vi "Compute alpha(beta) Plot.vi"(8 "Error In":errorcluster, 10 "Phasor Parameters":T1={"Display Parameters"={"# Points"=0, "Ramp Type"=enum."Linear", "Type of Series"=enum."1-Exp Decays", "Min tau"=0.0, "Max tau"=0.0, "Include 0"=FALSE, "Include Infinity"=FALSE}, "Phasor Parameters"={"Harmonic frequency"=0.0, "Use f* = 1/D Frequency"=FALSE, "Calibrated Phasor"=FALSE, "Calibration Lifetime"=1e-09, "Phasor Calculation"=enum."Direct Sum", "SEPL Type"=enum."UC", "# Gates"=1.0, "Square Gate Width"=1e-09, "Show Ticks"=FALSE}, "Decay & IRF Parameters"={"Lifetime"=0.0, "IRF Offset"=0.0, "Laser Period"=0.0, "Normalized Decays"=FALSE, "IRF Model"=enum."Dirac", "IRF Parameter 1"=0.0}, "Gate Parameters"={"First Gate Start"=0.0, "Use Gate Center"=FALSE, "Gate Width"=0.0, "Gate Step"=0.0, "# Gates"=0.0, "Gate Type"=enum."Square", "Edge Width"=0.0, "Top Slope"=0.0, "Reversed Sawtooth?"=FALSE, "Analytical Computation"=FALSE, "Tolerance"=1.0, "Integration"=enum."Item 0", "# Steps"=1.0, "Type of User-defined Function"=enum."Gate"}, "Detector Parameters"={"Frames/Image"=0, "Gates/Frame"=0, "Bits/Frame"=0, "Multiplicity"=0, "Incident Signal"=0.0}} {"Detector Parameters"."Frames/Image" min=1; "Detector Parameters"."Multiplicity" min=0; "Detector Parameters"."Bits/Frame" min=1; "Detector Parameters"."Gates/Frame" min=1; "Gate Parameters"."# Steps" min=0.0; "Gate Parameters"."Tolerance" min=0.0; "Gate Parameters"."Top Slope" min=0.0; "Gate Parameters"."Edge Width" min=0.0; "Gate Parameters"."Gate Step" min=0.0; "Gate Parameters"."# Gates" min=0.0 step=1.0; "Gate Parameters"."Gate Width" min=0.0; "Decay & IRF Parameters"."Lifetime" min=0.0; "Decay & IRF Parameters"."Laser Period" min=0.0; "Phasor Parameters"."Square Gate Width" min=0.0; "Phasor Parameters"."# Gates" min=0.0; "Phasor Parameters"."Calibration Lifetime" min=0.0; "Phasor Parameters"."Harmonic frequency" min=0.0; "Display Parameters"."Min tau" min=0.0; "Display Parameters"."Max tau" min=0.0; "Display Parameters"."# Points" min=1 step=1}, 11 "alpha(beta) Graph Refnum":refnum<vi>) -> (0 "Error Out":errorcluster, 2 "Max Lifetime":dbl[unit], 3 "Min Lifetime":dbl[unit])   [LabVIEW 2019]
uses:
  Pseudo Phasor Parameters.ctl
  Phasor Explorer Display Parameters.ctl
  Type of Series.ctl
  Phasor Explorer Phasor Parameters.ctl
  Phasor Calculation Type.ctl
  Phasor Type.ctl
  Phasor Explorer Decay Parameters.ctl
  IRF Model.ctl
  Phasor Explorer Gate Parameters.ctl
  Gate Type.ctl
  Phasor Explorer Detector Parameters.ctl
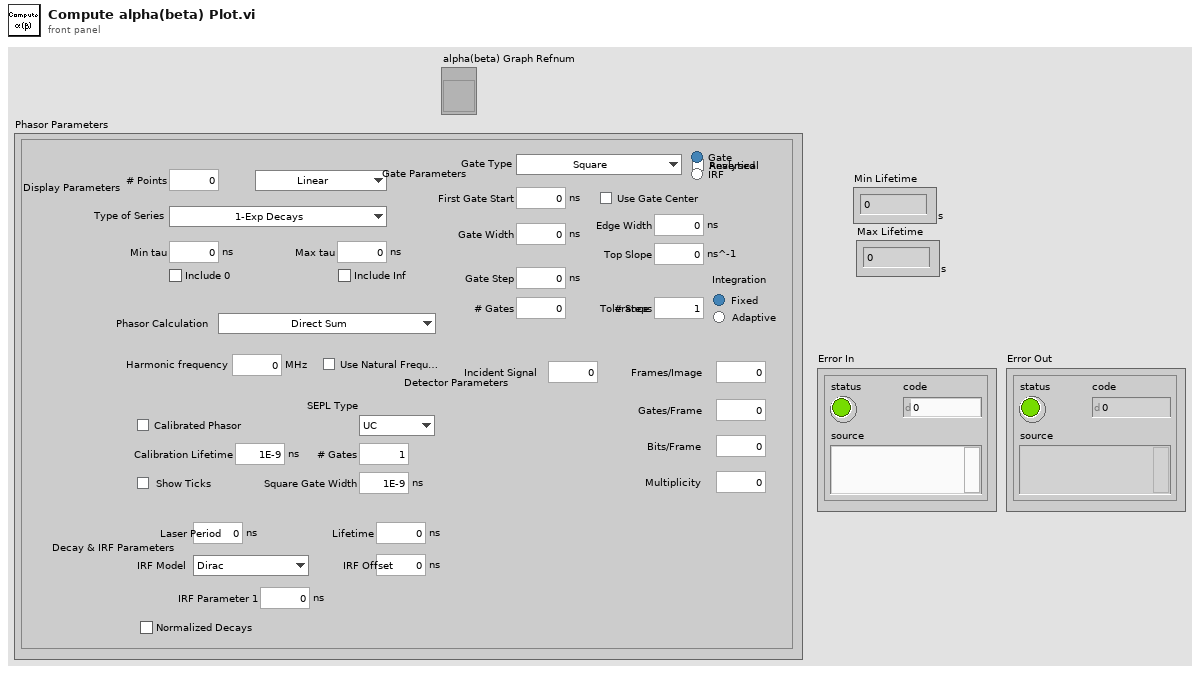
[diagram p1: front panel]
types:
  T1 = typedef "Pseudo Phasor Parameters.ctl" = cluster{"Display Parameters":T2, "Phasor Parameters":T4, "Decay & IRF Parameters":T7, "Gate Parameters":T9, "Detector Parameters":T11}
  T2 = typedef "Phasor Explorer Display Parameters.ctl" = cluster{"# Points":i32, "Ramp Type":enum16{"Linear", "Logarithmic"}, "Type of Series":T3, "Min tau":dbl[unit], "Max tau":dbl[unit], "Include 0":bool, "Include Infinity":bool}
  T3 = typedef "Type of Series.ctl" = enum16{"1-Exp Decays", "Linear Combination of 1-Exp"}
  T4 = typedef "Phasor Explorer Phasor Parameters.ctl" = cluster{"Harmonic frequency":dbl[unit], "Use f* = 1/D Frequency":bool, "Calibrated Phasor":bool, "Calibration Lifetime":dbl[unit], "Phasor Calculation":T5, "SEPL Type":T6, "# Gates":dbl, "Square Gate Width":dbl[unit], "Show Ticks":bool}
  T5 = typedef "Phasor Calculation Type.ctl" = enum16{"Direct Sum", "Analytical Formula"}
  T6 = typedef "Phasor Type.ctl" = enum16{"UC", "L_N", "L_N[W]"}
  T7 = typedef "Phasor Explorer Decay Parameters.ctl" = cluster{"Lifetime":dbl[unit], "IRF Offset":dbl[unit], "Laser Period":dbl[unit], "Normalized Decays":bool, "IRF Model":T8, "IRF Parameter 1":dbl[unit]}
  T8 = typedef "IRF Model.ctl" = enum16{"Dirac", "Exponential"}
  T9 = typedef "Phasor Explorer Gate Parameters.ctl" = cluster{"First Gate Start":dbl[unit], "Use Gate Center":bool, "Gate Width":dbl[unit], "Gate Step":dbl[unit], "# Gates":dbl, "Gate Type":T10, "Edge Width":dbl[unit], "Top Slope":dbl[unit], "Reversed Sawtooth?":bool, "Analytical Computation":bool, "Tolerance":dbl, "Integration":enum32{"Item 0", "Item 1"}, "# Steps":dbl, "Type of User-defined Function":enum32{"Gate", "IRF"}}
  T10 = typedef "Gate Type.ctl" = enum16{"Square", "Finite Edge Square", "Finite Edge, Tilted Top Square", "Triangle", "Sawtooth", "User-defined"}
  T11 = typedef "Phasor Explorer Detector Parameters.ctl" = cluster{"Frames/Image":i32, "Gates/Frame":i32, "Bits/Frame":i32, "Multiplicity":i32, "Incident Signal":dbl}
  T12 = typedef "Gate Definitions.ctl" = cluster{"First Gate: t1":ext, "Gate Width: W":ext, "Gate Step: d":ext, "# Gates: G":ext, "Use Gate Center":bool, "Frames/Image: F":i32, "Gates/Frame: L":i32, "Bits/Frame: q":i32, "Multiplicity: p":i32, "Gate Type":T10, "Gate Edge s":ext, "Gate Top Slope":ext, "Reversed Sawtooth?":bool, "Computation":bool, "User-defined Gate":T13, "Tolerance":ext, "Integration":enum32{"Item 0", "Item 1"}, "# Steps":ext, "Type of User-defined Function":enum32{"Gate", "IRF"}}
  T13 = typedef "XY Plot Data.ctl" = cluster{"X Array":dbl[], "Y Array":dbl[]}
  T14 = typedef "Decay Definiton.ctl" = cluster{"offset: t0":ext, "period: T":ext, "lifetime: tau":ext, "Incident Signal: I":ext, "Normalized Decays":bool, "IRF Model":T8, "IRF Parameter 1":ext}
  T15 = typedef "Phasor (g, s).ctl" = cluster{"g":dbl, "s":dbl}
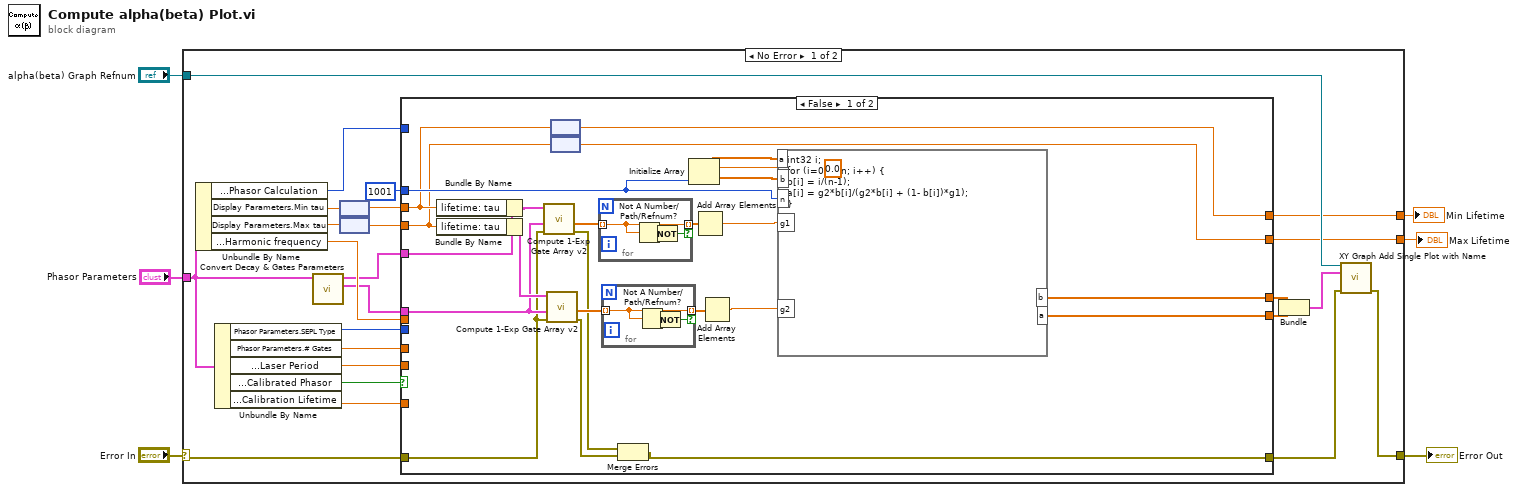
[diagram p0: block diagram]
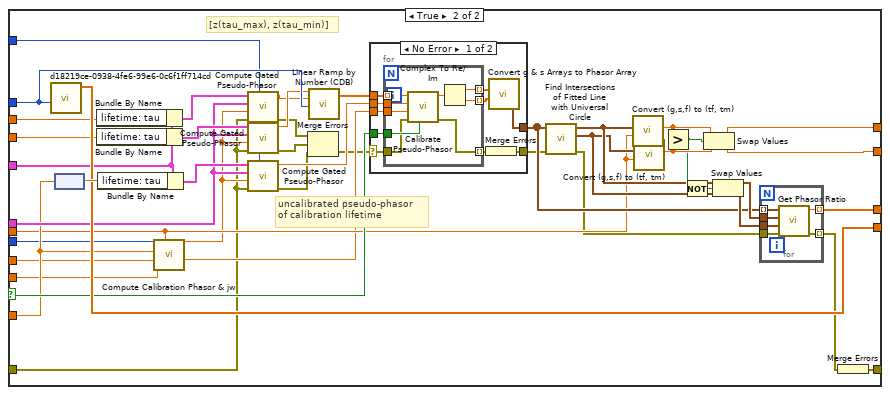
[diagram p2: hidden frame]
diagram:
  n1 = case shown="No Error" "Error In" {
    selector: "Error In" -> [w8 w130]
    tunnel: "Phasor Parameters" -> [w15 _]
    tunnel: "alpha(beta) Graph Refnum" -> [w28 _]
    tunnel: [w27 w130] -> w3
    tunnel: [w19 _] -> w2
    tunnel: [w18 _] -> w1
    frame No Error {
      n2 = Unbundle By Name(w15) -> ("Phasor Parameters.Phasor Calculation"=w12:T5, "Display Parameters.Min tau"=w29:dbl[unit], "Display Parameters.Max tau"=w30:dbl[unit], "Phasor Parameters.Harmonic frequency"=w20:dbl[unit])
      n3 = Unbundle By Name(w15) -> ("Phasor Parameters.SEPL Type"=w11:T6, "Phasor Parameters.# Gates"=w10:dbl, "Decay & IRF Parameters.Laser Period"=w9:dbl[unit], "Phasor Parameters.Calibrated Phasor"=w14:bool, "Phasor Parameters.Calibration Lifetime"=w13:dbl[unit])
      n4 = call "Convert Decay & Gates Parameters.vi"("Phasor Parameters"=w15) -> ("Gates Definitions"=w16:T12, "Decay Definition"=w17:T14)  [unwired: 9 in]
      n5 = node(w29) -> (w25:dbl)
      n6 = node(w30) -> (w24:dbl)
      n7 = case shown="False" w14 {
        selector: w14 -> [_ w80]
        tunnel: w17 -> [w52 w88]
        tunnel: w25 -> [w42 w89]
        tunnel: w24 -> [w40 w87]
        tunnel: w16 -> [w50 w84]
        tunnel: [w45 w91] -> w23
        tunnel: [w44 w90] -> w22
        tunnel: 1001 ("dimension size") -> [w43 w83]
        tunnel: w20 -> [_ w74]
        tunnel: [w41 w99] -> w19
        tunnel: [w39 w98] -> w18
        tunnel: w13 -> [_ w75]
        tunnel: w12 -> [_ w76]
        tunnel: w11 -> [_ w72]
        tunnel: w10 -> [_ w71]
        tunnel: w9 -> [_ w70]
        tunnel: w8 -> [w34 w68]
        tunnel: [w32 w62] -> w7
        frame False {
          n8 = Bundle By Name(cluster=w52, "lifetime: tau"=w42) -> (w51:T14)
          n9 = Bundle By Name(cluster=w52, "lifetime: tau"=w40) -> (w53:T14)
          n10 = call "Compute 1-Exp Gate Array v2.vi"("Error In"=w34, "Gates Definitions"=w50, "Decay Definition"=w51) -> ("Error Out"=w31:errorcluster, "Gate Image Array"=w38:ext[])  [unwired: 4 in, 3 out]
          n11 = call "Compute 1-Exp Gate Array v2.vi"("Error In"=w34, "Gates Definitions"=w50, "Decay Definition"=w53) -> ("Error Out"=w33:errorcluster, "Gate Image Array"=w36:ext[])  [unwired: 4 in, 3 out]
          n12 = node(w42) -> (w41:dbl[unit])
          n13 = node(w40) -> (w39:dbl[unit])
          n14 = for {
            tunnel: w38 -> [w59] mode=indexing
            tunnel: [w59] -> w37 mode=indexing if=w57
            n15 = Not A Number/Path/Refnum?(number/path/refnum=w59) -> (NaN/Path/Refnum?=w58:bool)
            n16 = Not(x=w58) -> (.not. x?=w57:bool)
          }
          n17 = for {
            tunnel: w36 -> [w56] mode=indexing
            tunnel: [w56] -> w35 mode=indexing if=w54
            n18 = Not A Number/Path/Refnum?(number/path/refnum=w56) -> (NaN/Path/Refnum?=w55:bool)
            n19 = Not(x=w55) -> (.not. x?=w54:bool)
          }
          n20 = Merge Errors(w31, w33) -> (w32:errorcluster)
          n21 = Initialize Array(0.0 ("element"), w43) -> (w46:dbl[])
          n22 = Add Array Elements(numeric array=w37) -> (sum=w49:ext)
          n23 = Add Array Elements(numeric array=w35) -> (sum=w48:ext)
          n24 = formula code="int32 i;\nfor (i=0; i<n; i++) {\nb[i] = i/(n-1);\na[i] = g2*b[i]/(g2*b[i] + (1- b[i])*g1);\n}"("g1"=w49, "g2"=w48, "b"=w46, "a"=w46, "n"=w43) -> ("b"=w45:dbl[], "a"=w44:dbl[])
        }
        frame True {
          # "[z(tau_max), z(tau_min)]"
          # "uncalibrated pseudo-phasor\nof calibration lifetime"
          n25 = call "d18219ce-0938-4fe6-99e6-0c6f1ff714cd.vi"("# Steps (1)"=w83) -> ("Ramp"=w90:dbl[])  [unwired: 9 in, 1 out]
          n26 = node(w75) -> (w102:dbl)
          n27 = Bundle By Name(cluster=w88, "lifetime: tau"=w89) -> (w86:T14)
          n28 = Bundle By Name(cluster=w88, "lifetime: tau"=w87) -> (w85:T14)
          n29 = Bundle By Name(cluster=w88, "lifetime: tau"=w102) -> (w103:T14)
          n30 = call "Compute Calibration Phasor & jw.vi"("Harmonic frequency"=w74, "Laser Period"=w70, "# Gates"=w71, "Calibration Lifetime"=w75, "Calibration Phasor Type"=w72) -> ("z (tau_cal)"=w69:cdb, "i 2 pi f (GHz)"=w73:cdb)  [unwired: 5 in]
          n31 = call "Compute Gated Pseudo-Phasor.vi"("Phasor Calculation Type"=w76, "Error In"=w68, "j 2 pi f"=w73, "Gates Definitions"=w84, "Decay Definition"=w86) -> ("Error Out"=w67:errorcluster, "phasor"=w78:cxt)  [unwired: 4 in, 1 out]
          n32 = call "Compute Gated Pseudo-Phasor.vi"("Phasor Calculation Type"=w76, "Error In"=w68, "j 2 pi f"=w73, "Gates Definitions"=w84, "Decay Definition"=w85) -> ("Error Out"=w66:errorcluster, "phasor"=w79:cxt)  [unwired: 4 in, 1 out]
          n33 = call "Compute Gated Pseudo-Phasor.vi"("Phasor Calculation Type"=w76, "Error In"=w68, "j 2 pi f"=w73, "Gates Definitions"=w84, "Decay Definition"=w103) -> ("Error Out"=w65:errorcluster, "phasor"=w81:cxt)  [unwired: 4 in, 1 out]
          n34 = Merge Errors(w67, w66, w65) -> (w61:errorcluster)
          n35 = call "Linear Ramp by Number (CDB).vi"("# Steps"=w83, "End"=w78, "Start"=w79) -> ("Ramp"=w82:cdb[])  [unwired: 7 in, 1 out]
          n36 = case shown="No Error" w61 {
            selector: w61 -> [w106 w123]
            tunnel: [w113 _] -> w92
            tunnel: w82 -> [w112 _]
            tunnel: w81 -> [w111 _]
            tunnel: w80 -> [w108 _]
            tunnel: w69 -> [w107 _]
            tunnel: [w104 w123] -> w60
            frame No Error {
              n37 = for {
                tunnel: w112 -> [w121] mode=indexing
                tunnel: w111 -> [w120]
                tunnel: w107 -> [w119]
                tunnel: [w118] -> w110 mode=indexing
                tunnel: [w117] -> w109 mode=indexing
                tunnel: w108 -> [w116]
                tunnel: w106 -> [w115]
                tunnel: [w114] -> w105 mode=indexing
                n38 = call "Calibrate Pseudo-Phasor.vi"("Calibrated Phasor"=w116, "Error In"=w115, "Target Phasor"=w119, "Calibration Pseudo-Phasor"=w120, "Pseudo-Phasor in"=w121) -> ("Error Out"=w114:errorcluster, "Pseudo-Phasor out"=w122:cxt)  [unwired: 5 in]
                n39 = Complex To Re/Im(x + iy=w122) -> (x=w118:ext, y=w117:ext)
              }
              n40 = Merge Errors(w105) -> (w104:errorcluster)
              n41 = call "Convert g & s Arrays to Phasor Array.vi"("s"=w109, "g"=w110) -> ("Phasor Array"=w113:T15[])  [unwired: 8 in]
            }
            frame Error {
            }
          }
          n42 = call "Find Intersections of Fitted Line with Universal Circle.vi"("Error In"=w60, "Phasor Array"=w92) -> ("Error Out"=w64:errorcluster, "Point 2"=w95:cluster{"x":dbl, "y":dbl}, "Point 1"=w96:cluster{"x":dbl, "y":dbl})  [unwired: 7 in]
          n43 = call "Convert (g,s,f) to (tf, tm).vi"("Phasor Harmonic Frequency"=w74, "Phasor (g, s)"=w96) -> ("Phase Lifetime"=w101:dbl[unit])  [unwired: 8 in, 1 out]
          n44 = call "Convert (g,s,f) to (tf, tm).vi"("Phasor Harmonic Frequency"=w74, "Phasor (g, s)"=w95) -> ("Phase Lifetime"=w100:dbl[unit])  [unwired: 8 in, 1 out]
          n45 = Greater?(x=w101, y=w100) -> (0:w97:bool)
          n46 = Not(x=w97) -> (.not. x?=w77:bool)
          n47 = Swap Values(12:w101, 13:w97, 14:w100) -> (1:w99:dbl[unit], 3:w98:dbl[unit])
          n48 = Swap Values(12:w96, 13:w77, 14:w95) -> (1:w94:cluster{"x":dbl, "y":dbl}, 3:w93:cluster{"x":dbl, "y":dbl})
          n49 = for {
            tunnel: w94 -> [w129]
            tunnel: w93 -> [w128]
            tunnel: w92 -> [w127] mode=indexing
            tunnel: [w126] -> w91 mode=indexing
            tunnel: w64 -> [w125]
            tunnel: [w124] -> w63 mode=indexing
            n50 = call "Get Phasor Ratio.vi"("Error In"=w125, "Reference Phasor 2"=w128, "Reference Phasor 1"=w129, "Phasor"=w127) -> ("Error Out"=w124:errorcluster, "Phasor Ratio"=w126:dbl)  [unwired: 6 in]
          }
          n51 = Merge Errors(w63) -> (w62:errorcluster)
        }
      }
      n52 = Bundle("b"=w23, "Ramp"=w22) -> (w26:cluster{"b":dbl[], "Ramp":dbl[]})  [unwired: 1 in]
      n53 = call "XY Graph Add Single Plot with Name.vi"("XYGraph Ref in"=w28, "Plot"=w26, "error in (no error)"=w7) -> ("error out"=w27:errorcluster)  [unwired: 9 in, 3 out]
    }
    frame Error {
    }
  }
  "Error Out" <- w3
  "Min Lifetime" <- w2
  "Max Lifetime" <- w1
